vi "실습 3-5 Running Average.vi"() -> ()   [LabVIEW 2014]
uses:
  <vilib>/ptbypt/NI_PtbyPt.lvlib
panel:
  in  "정지":bool
  out "웨이브폼 차트":cluster{dbl, dbl, "mean":dbl}(graph)
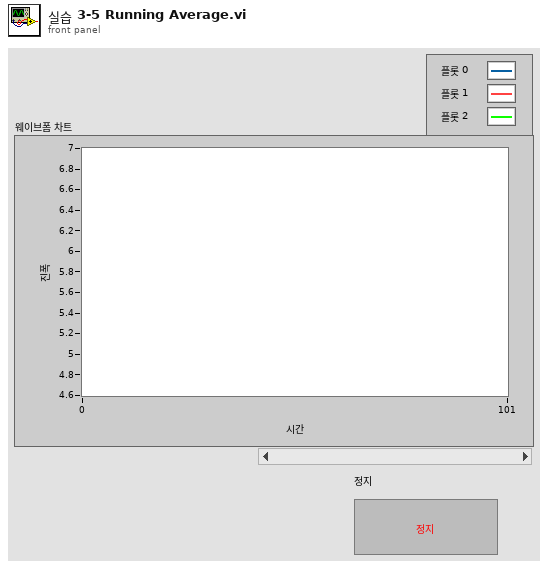
[diagram p1: front panel]
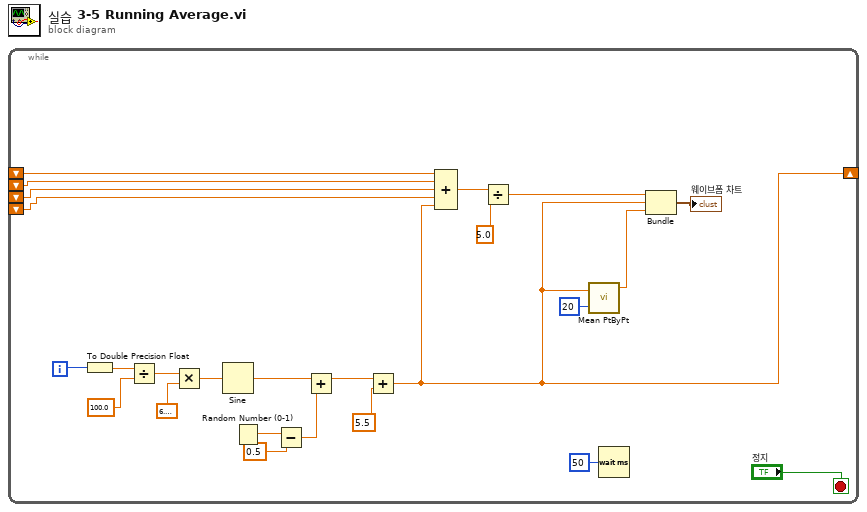
[diagram p0: block diagram]
diagram:
  n1 = while {
    shift-right: [w3] -> _
    shift-left: _ -> [w11]
    shift-left: _ -> [w10]
    shift-left: _ -> [w9]
    shift-left: _ -> [w8]
    i -> [w23]
    stop <- "정지" stop-if-true
    n2 = To Double Precision Float(number=w23) -> (double precision float=w22:dbl)
    n3 = Divide(x=w22, y=100.0) -> (x/y=w20:dbl)
    n4 = Multiply(x=w20, y=6.283185307179586) -> (x*y=w18:dbl)
    n5 = Sine(x=w18) -> (sin(x)=w17:dbl)
    n6 = Random Number (0-1)() -> (number: 0 to 1=w16:dbl)
    n7 = Subtract(x=w16, y=0.5) -> (x-y=w13:dbl)
    n8 = Add(x=w17, y=w13) -> (x+y=w14:dbl)
    n9 = Add(x=w14, y=5.5) -> (x+y=w3:dbl)
    n10 = Compound Arithmetic op=ADD(w11, w10, w9, w8, w3) -> (w7:dbl)
    n11 = Divide(x=w7, y=5.0) -> (x/y=w5:dbl)
    n12 = call <vilib>:"Mean PtByPt.vi"("x"=w3, "sample length"=20) -> ("mean"=w1:dbl)  [unwired: 2 in, 1 out]
    n13 = Wait (ms)(milliseconds to wait=u32 50 ("대기 시간(ms)")) -> ()  [unwired: 1 out]
    n14 = Bundle(w5, w3, "mean"=w1) -> (→"웨이브폼 차트":cluster{dbl, dbl, "mean":dbl})  [unwired: 1 in]
  }
